vi "SetIndex.vi"(0 "reference in":refnum<class "MusicPlayer.lvclass">, 7 "Index":u32, 11 "Error In":errorcluster) -> (4 "reference out":refnum<class "MusicPlayer.lvclass">, 15 "Error Out":errorcluster)   [LabVIEW 2022 SP3, in "MusicPlayer.lvclass"]
uses:
  MusicPlayer.lvclass
  MusicPlayer.lvclass/MusicPlayer.ctl
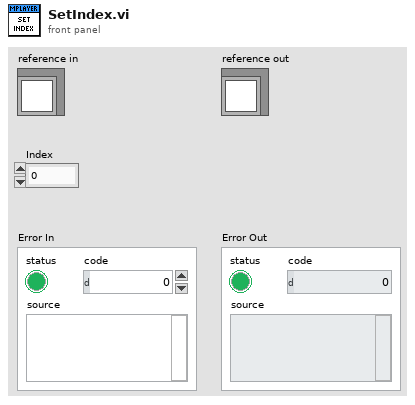
[diagram p1: front panel]
types:
  T1 = typedef "MusicPlayer.lvclass/ObjectAttributes.ctl" = cluster{"MediaPlayer":refnum<k7>, "Playlist":path[], "Index":u32}
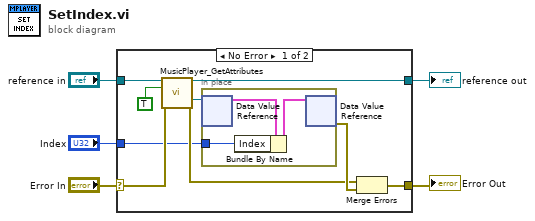
[diagram p0: block diagram]
diagram:
  n1 = case shown="No Error" "Error In" {
    selector: "Error In" -> [w12 w19]
    tunnel: [w7 w19] -> w4
    tunnel: [w13 w18] -> w2
    tunnel: "reference in" -> [w14 w18]
    tunnel: "Index" -> [w6 _]
    frame No Error {
      n2 = call "MusicPlayer_GetAttributes.vi"("reference in"=w14, "OnlyGetDvrReference(False)"=TRUE, "error in (no error)"=w12) -> ("reference out"=w13:refnum<class "MusicPlayer.lvclass">, "DataRef"=w9:refnum<data-value>, "error out"=w8:errorcluster)  [unwired: 9 in, 1 out]
      n3 = in-place {
        in-place-border: w6 -> [w17]
        n4 = in-place-dvr #1(w9) -> (w16:T1)  [unwired: 1 out]
        n5 = Bundle By Name(cluster=w16, "Index"=w17) -> (w15:T1)
        n6 = in-place-dvr #1(w15) -> (w10:errorcluster)  [unwired: 1 out]
      }
      n7 = Merge Errors(w8, w10) -> (w7:errorcluster)
    }
    frame Error {
    }
  }
  "Error Out" <- w4
  "reference out" <- w2
